vi "Get Wavelength.vi"(8 "error in":errorcluster, 11 "reference":refnum<k24>) -> (0 "error out":errorcluster, 2 "GetOutputWavelength":dbl, 3 "reference out":refnum<k24>)   [LabVIEW 2020, in "Topas4.lvlib"]
uses:
  Topas4.lvlib
  C:/Windows/SysWOW64/Topas4Lib.dll
  Windows/SysWOW64/Topas4Lib.dll
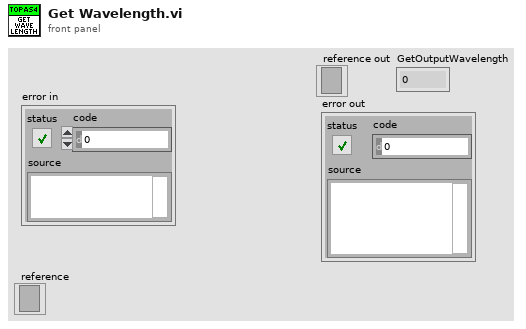
[diagram p1: front panel]
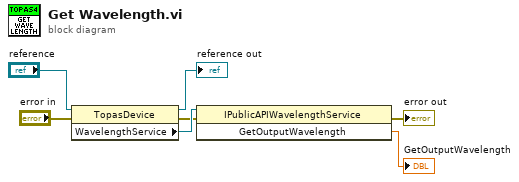
[diagram p0: block diagram]
diagram:
  n1 = property class="TopasDevice"(reference="reference", error in="error in") -> (reference out=→"reference out":refnum<k24>, error out=w3:errorcluster, "WavelengthService"=w4:refnum<k24>)
  n2 = invoke class="IPublicAPIWavelengthService" method="GetOutputWavelength"(reference=w4, error in=w3) -> (error out=→"error out":errorcluster, "GetOutputWavelength"=→"GetOutputWavelength":dbl)  [unwired: 1 in, 1 out]
